vi "UI_Find Selected History icon.vi"(7 "Border Size":i32=4, 8 "Error":errorcluster, 9 "Mouse Cord":T1, 11 "Array REf":refnum<vi>) -> (0 "Error Out":errorcluster, 1 "Valid Out":bool, 2 "Index Out":i32, 3 "Array REf Out":refnum<vi>)   [LabVIEW 2009]
doc: "Find Index of selected array item from mouse position"
uses:
  Controls/Cluster/Cluster_Mouse Location.ctl
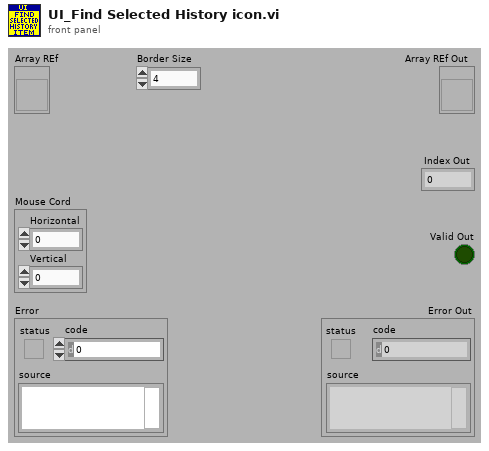
[diagram p1: front panel]
types:
  T1 = typedef "Cluster_Mouse Location.ctl" = cluster{"Horizontal":i32, "Vertical":i32}
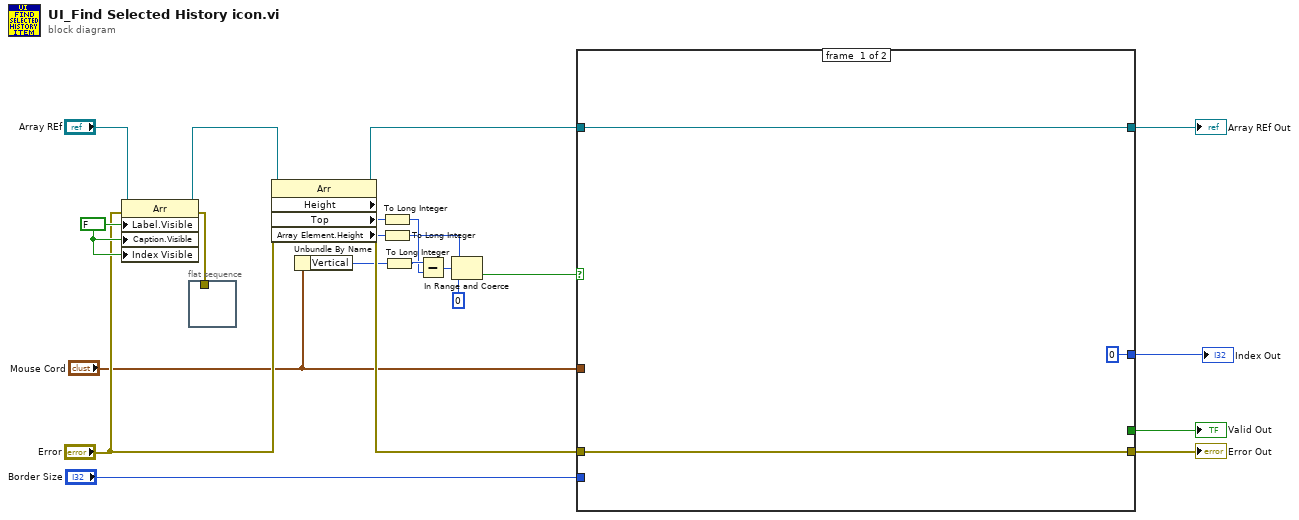
[diagram p0: block diagram]
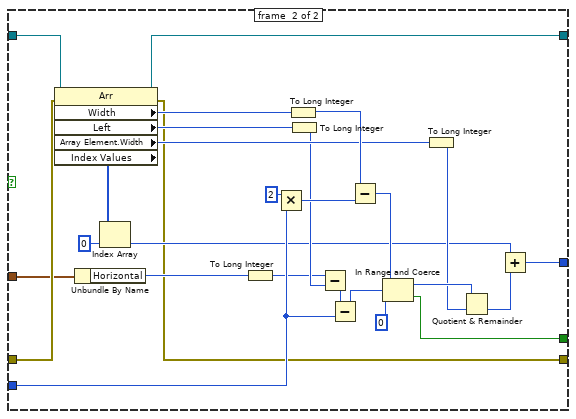
[diagram p2: hidden frame]
diagram:
  w21 = FALSE ("Label.Visible")
  n1 = property class="Arr"(reference="Array REf", error in="Error", "Label.Visible"=w21, "Caption.Visible"=w21, "Index Visible"=w21) -> (reference out=w12:refnum<vi>, error out=w15:errorcluster)
  n2 = flat-sequence {
    tunnel: w15 -> [_]
    frame #0 {
    }
  }
  n3 = property class="Arr" props=["Height", "Top", "Array Element", "Height"](reference=w12, error in="Error") -> (reference out=w11:refnum<vi>, error out=w13:errorcluster, "Top"=w9:i32, "Array Element.Height"=w8:u32)  [unwired: 1 out]
  n4 = Unbundle By Name("Mouse Cord") -> ("Vertical"=w7:i32)
  n5 = To Long Integer(number=w9) -> (32bit integer=w5:i32)
  n6 = To Long Integer(number=w8) -> (32bit integer=w3:i32)
  n7 = To Long Integer(number=w7) -> (32bit integer=w6:i32)
  n8 = Subtract(x=w6, y=w5) -> (x-y=w1:i32)
  n9 = In Range and Coerce(upper limit=w3, x=w1, lower limit=0) -> (In Range?=w2:bool)  [unwired: 1 out]
  n10 = case shown="False" w2 {
    tunnel: "Border Size" -> [_ w41]
    tunnel: [_ w36] -> w19
    tunnel: [w25 w33] -> w18
    tunnel: [w23 w32] -> w17
    tunnel: [u32 0 w31] -> w16
    tunnel: w13 -> [w25 w30]
    tunnel: w11 -> [w23 w29]
    tunnel: "Mouse Cord" -> [_ w28]
    frame #0 {
    }
    frame #1 {
      n11 = property class="Arr"(reference=w29, error in=w30) -> (reference out=w32:refnum<vi>, error out=w33:errorcluster, "Width"=w48:u32, "Left"=w47:i32, "Array Element.Width"=w40:u32, "Index Values"=w27:u32[])
      n12 = Unbundle By Name(w28) -> ("Horizontal"=w44:i32)
      n13 = Index Array(array=w27, index=0) -> (element=w35:u32)
      n14 = To Long Integer(number=w44) -> (32bit integer=w38:i32)
      n15 = Multiply(x=2, y=w41) -> (x*y=w43:i32)
      n16 = To Long Integer(number=w48) -> (32bit integer=w52:i32)
      n17 = To Long Integer(number=w47) -> (32bit integer=w39:i32)
      n18 = Subtract(x=w38, y=w39) -> (x-y=w45:i32)
      n19 = Subtract(x=w45, y=w41) -> (x-y=w46:i32)
      n20 = Subtract(x=w52, y=w43) -> (x-y=w49:i32)
      n21 = In Range and Coerce(upper limit=w49, x=w46, lower limit=0) -> (coerced(x)=w51:i32, In Range?=w36:bool)
      n22 = To Long Integer(number=w40) -> (32bit integer=w37:i32)
      n23 = Quotient & Remainder(x=w51, y=w37) -> (floor(x/y)=w34:i32)  [unwired: 1 out]
      n24 = Add(x=w35, y=w34) -> (x+y=w31:u32)
    }
  }
  "Index Out" <- w16
  "Error Out" <- w18
  "Valid Out" <- w19
  "Array REf Out" <- w17
